vi "JoinWorksheets.vi"(8 "error in (no error)":errorcluster, 10 "ExcelFile To Join":refnum<class "PortableExcelFileManipulationOXML.lvclass">, 11 "ExcelFile in":refnum<class "PortableExcelFileManipulationOXML.lvclass">) -> (0 "error out":errorcluster, 3 "ExcelFile out":refnum<class "PortableExcelFileManipulationOXML.lvclass">)   [LabVIEW 2019, in "PortableExcelFileManipulationOXML.lvclass"]
doc: "Adds a worksheet to the This excel File by name."
uses:
  PortableExcelFileManipulationOXML.lvclass
  PortableExcelFileManipulationOXML.lvclass/PortableExcelFileManipulationOXML.ctl
  H:/LV projects/ExpressionEvaluator/Excel/ExcelManipulation.dll
  ExcelManipulation.dll
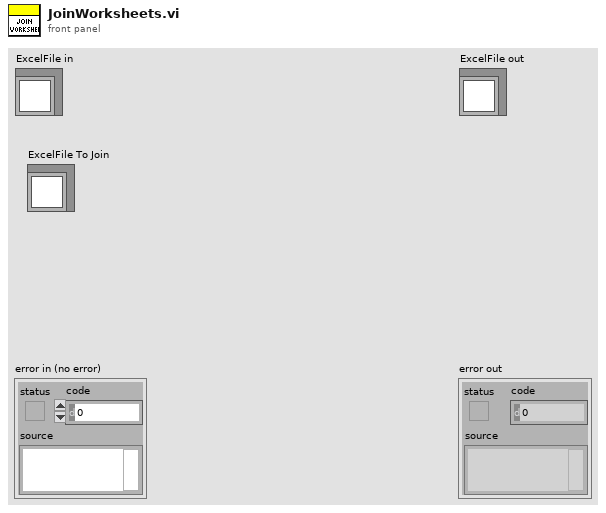
[diagram p1: front panel]
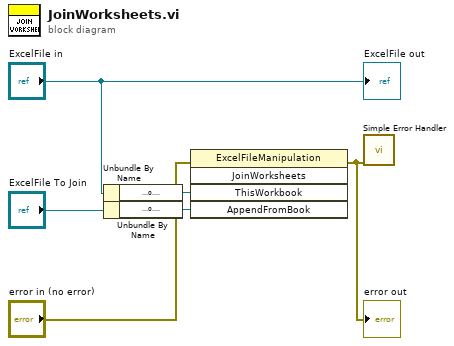
[diagram p0: block diagram]
diagram:
  n1 = Unbundle By Name("ExcelFile in") -> ("ExcelOpen"=w4:refnum<k24>)
  n2 = Unbundle By Name("ExcelFile To Join") -> ("ExcelOpen"=w3:refnum<k24>)
  n3 = invoke class="ExcelFileManipulation" method="JoinWorksheets"(error in="error in (no error)", "ThisWorkbook"=w4, "AppendFromBook"=w3) -> (error out=w1:errorcluster)  [unwired: 2 in, 4 out]
  "error out" <- w1
  n4 = call <vilib>:"Simple Error Handler.vi"("error in (no error)"=w1) -> ()  [unwired: 4 in, 5 out]
  "ExcelFile out" <- "ExcelFile in"
